vi "FlatToRichGreeter_req.vi"(5 "OutputClusterType":T1, 11 "InputCluster":T3) -> (3 "OutputCluster":T1)   [LabVIEW 2019, in "Generated_server.lvlib"]
uses:
  Generated_server.lvlib
  Greeter_req_Flat.ctl
  Greeter_MessageA_Flat.ctl
  Greeter_req.ctl
  Greeter_req_req_oneof/Greeter_req_req_oneof.lvclass
  Greeter_MessageA.ctl
  Greeter_req_req_oneof/Greeter_req_req_oneof.lvclass/Greeter_req_req_oneof.ctl
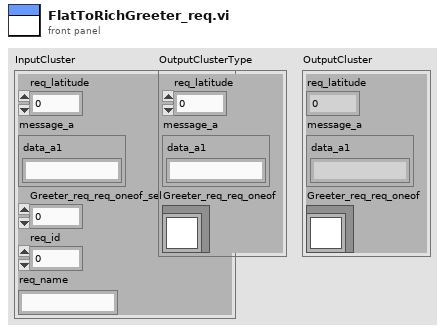
[diagram p1: front panel]
types:
  T1 = typedef "Generated_server.lvlib/Greeter_req.ctl" = cluster{"req_latitude":i32, "message_a":T2, "Greeter_req_req_oneof":refnum<class "Greeter_req_req_oneof.lvclass">}
  T2 = typedef "Generated_server.lvlib/Greeter_MessageA.ctl" = cluster{"data_a1":string}
  T3 = typedef "Generated_server.lvlib/Greeter_req_Flat.ctl" = cluster{"req_latitude":i32, "message_a":T4, "Greeter_req_req_oneof_selected_index":i32, "req_id":i32, "req_name":string}
  T4 = typedef "Generated_server.lvlib/Greeter_MessageA_Flat.ctl" = cluster{"data_a1":string}
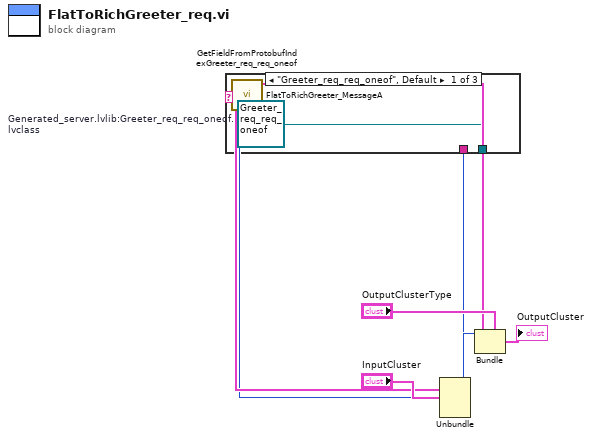
[diagram p0: block diagram]
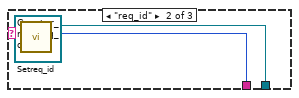
[diagram p2: hidden frame]
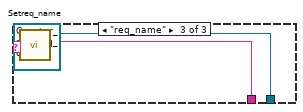
[diagram p3: hidden frame]
diagram:
  n1 = Unbundle "Unbundle"("InputCluster") -> ("req_latitude"=w8:i32, "message_a"=w7:T4, "Greeter_req_req_oneof_selected_index"=w5:i32, "req_id"=w2:i32, "req_name"=w1:string)
  n2 = call "GetFieldFromProtobufIndexGreeter_req_req_oneof.vi"("protobuf index"=w5) -> ("oneof field name"=w4:string)
  n3 = case "Greeter_req_req_oneof" shown="\"Greeter_req_req_oneof\", Default" w4 {
    tunnel: [w12 w14 w17] -> w3
    tunnel: w2 -> [_ w15 _]
    tunnel: w1 -> [_ _ w18]
    frame "Greeter_req_req_oneof", Default {
      w12 = refnum<class "Greeter_req_req_oneof.lvclass"> refnum  # Generated_server.lvlib:Greeter_req_req_oneof.lvclass
    }
    frame "req_id" {
      n4 = call "Setreq_id.vi"("Set_Val"=w15, "OneOfTemplate in"=refnum<class "Greeter_req_req_oneof.lvclass"> refnum) -> ("OneOfTemplate out"=w14:refnum<class "Greeter_req_req_oneof.lvclass">)  [unwired: 8 in, 1 out]
    }
    frame "req_name" {
      n5 = call "Setreq_name.vi"("Set_Val"=w18, "OneOfTemplate in"=refnum<class "Greeter_req_req_oneof.lvclass"> refnum) -> ("OneOfTemplate out"=w17:refnum<class "Greeter_req_req_oneof.lvclass">)  [unwired: 8 in, 1 out]
    }
  }
  n6 = call "FlatToRichGreeter_MessageA.vi"("InputCluster"=w7) -> ("OutputCluster"=w6:T2)  [unwired: 10 in]
  n7 = Bundle "Bundle"(cluster="OutputClusterType", "req_latitude"=w8, "message_a"=w6, "Greeter_req_req_oneof"=w3) -> (→"OutputCluster":T1)
